vi "Read Encoding.vi"(8 "error in (no error)":errorcluster, 11 "SQL Statement in":refnum<class "SQL Statement.lvclass">) -> (0 "error out":errorcluster, 2 "Encoding":T1, 3 "SQL Statement out":refnum<class "SQL Statement.lvclass">)   [LabVIEW 2013, in "SQLiteSupport.lvlib" / "SQL Statement.lvclass"]
doc: "Text encoding for string inputs or outputs, including SQL scripts. \n1) System -- Assumed to be the system encoding used by LabVIEW. Text is converted to UTF-8 before being passed to SQLite, and UTF-8 results from SQLite are coverted back the the system encoding.\n2) UTF-8 -- Strings assumed to be UTF-8. Note that ANSI, used by English Windows LabVIEW, is a valid subset of UTF-8.\n3) UTF-16 -- Strings assumed to be UTF-16.\n\nNote that encoding does not affect BLOB binary data."
uses:
  SQL Statement.lvclass
  SQL Statement.lvclass/SQL Statement.ctl
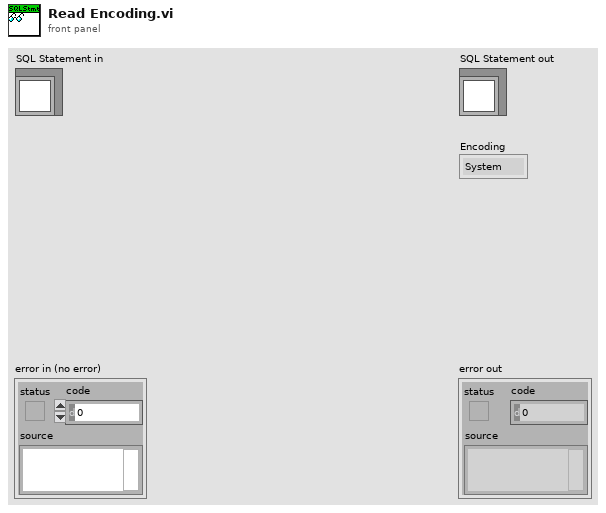
[diagram p1: front panel]
types:
  T1 = typedef "SQLiteSupport.lvlib/SQL Statement.lvclass/Text Encoding" = enum16{"System", "UTF-8", "UTF-16"}
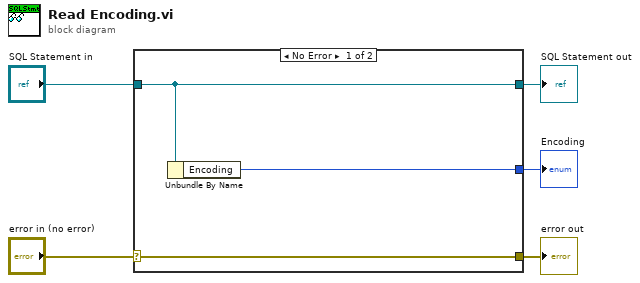
[diagram p0: block diagram]
diagram:
  n1 = case shown="No Error" "error in (no error)" {
    selector: "error in (no error)" -> [w8 w9]
    tunnel: [w8 w9] -> w4
    tunnel: [w7 w10] -> w2
    tunnel: "SQL Statement in" -> [w7 w10]
    tunnel: [w6 _] -> w1
    frame No Error {
      n2 = Unbundle By Name(w7) -> ("Encoding"=w6:T1)
    }
    frame Error {
    }
  }
  "error out" <- w4
  "SQL Statement out" <- w2
  "Encoding" <- w1
